vi "Send All HardWare Parameters Sending.vi"(0 "VISA resource name":refnum<visa-resource-name>="COM6", 5 "Corner Frecuency 1 [MHz]":u8=1 min=1 max=30 step=1, 7 "Corner Frecuency 2 [MHz]":u8=1 min=1 max=30 step=1, 9 "Gain VGA A (dB)":i8=-5 min=-5 max=45 step=1, 11 "Output Gain A":bool, 12 "Gain VGA B (dB)":i8=-5 min=-5 max=45 step=1, 13 "Output Gain B":bool) -> (10 "Coincidence Of Character":bool)   [LabVIEW 2011]
panel:
  in  "Numeric 3":fxp<+,12,12>
  out "String Sent DAC B":string
  out "Information Recieved DAC B":string
  out "Information Recieved DAC A":string
  out "String Sent DAC A":string
  in  "Numeric 2":fxp<+,12,12>
  out "Information Recieved PFVGA 2":string
  out "String Sent PFVGA 2":string
  out "Information Recieved PFVGA":string
  out "String Sent PFVGA":string
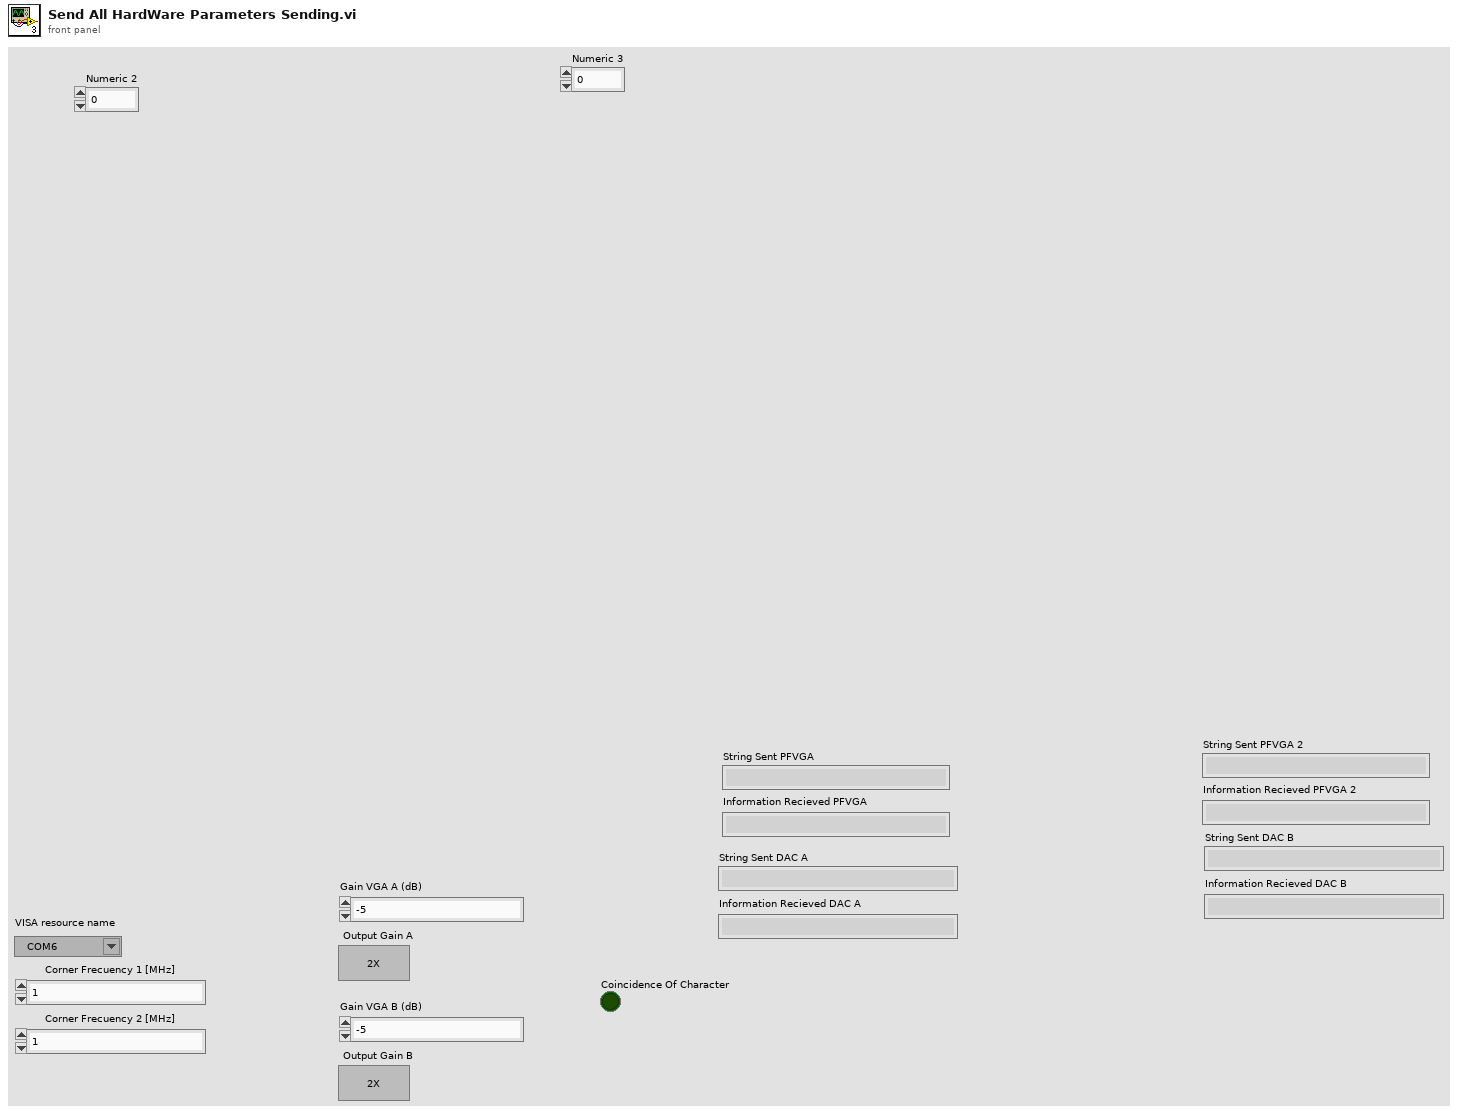
[diagram p1: front panel]
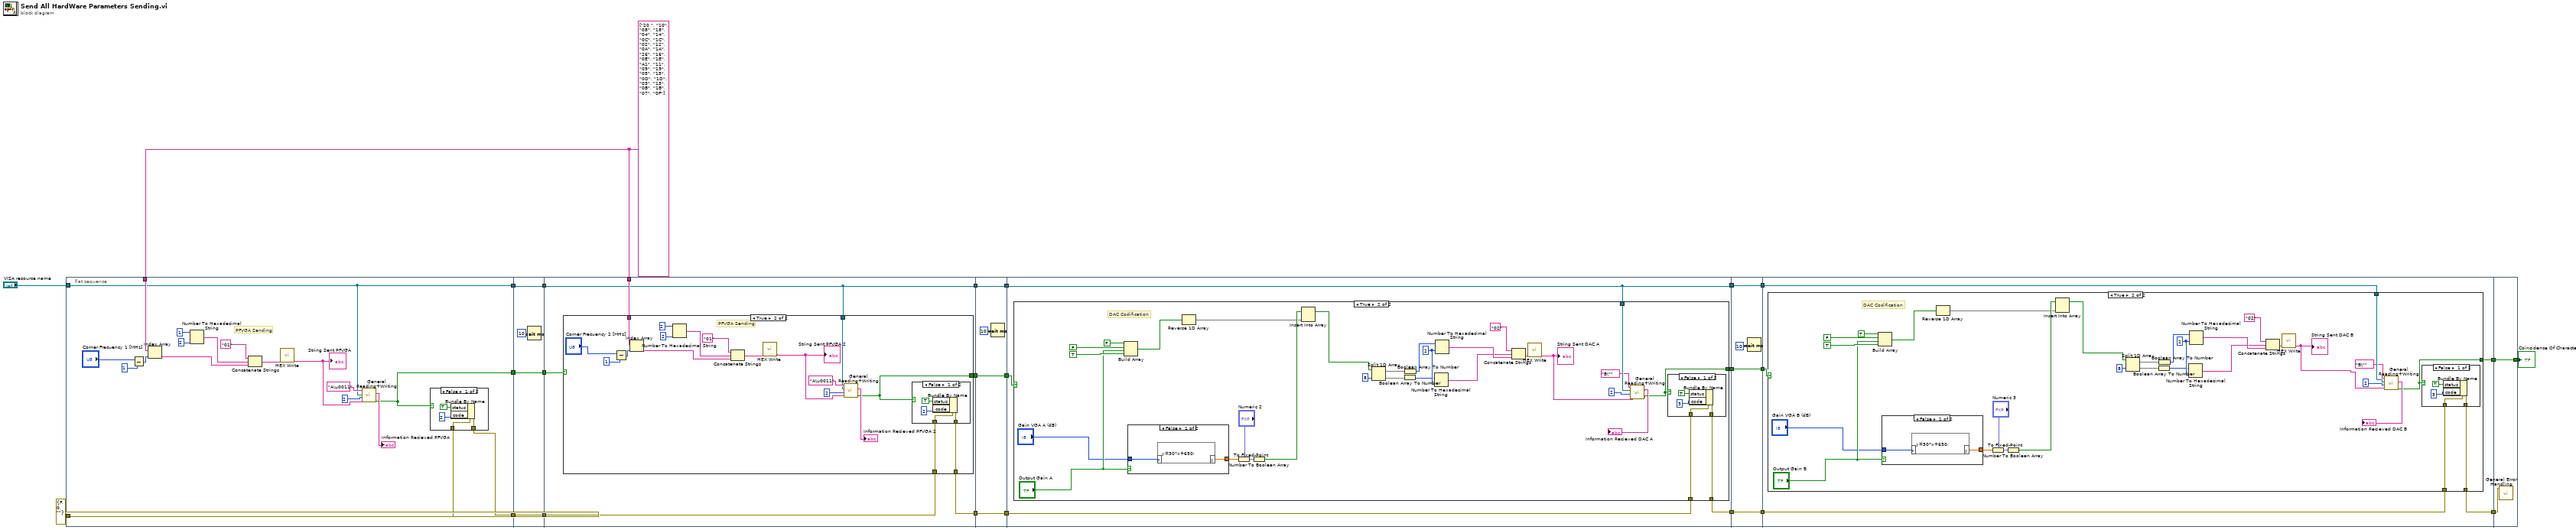
[diagram p0: block diagram]
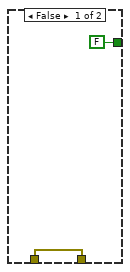
[diagram p3: hidden frame]
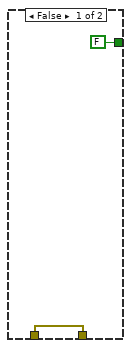
[diagram p5: hidden frame]
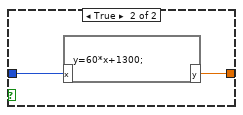
[diagram p7: hidden frame]
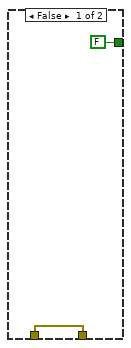
[diagram p8: hidden frame]
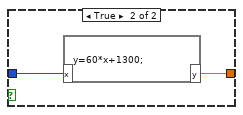
[diagram p10: hidden frame]
diagram:
  w23 = string[] ["20 ", "10", "08", "18", "04", "14", "0C", "1C", "02", "12", "0A", "1A", "26", "16", "0E", "1E", "A1", "11", "09", "19", "05", "15", "0D", "1D", "03", "13", "0B", "1B", "07", "0F"] ("Array")
  n1 = flat-sequence {
    tunnel: w23 -> [w33]
    tunnel: errorcluster {"status"=FALSE, "code"=0, "source"=""} ("error out") -> [w32]
    tunnel: [w31] -> w18
    tunnel: "VISA resource name" -> [w27]
    tunnel: [w25] -> w16
    tunnel: [w27] -> w14
    tunnel: w18 -> [w51]
    tunnel: [w51] -> w17
    tunnel: w16 -> [w50]
    tunnel: [w50] -> w15
    tunnel: w14 -> [w49]
    tunnel: [w49] -> w13
    tunnel: w17 -> [w56]
    tunnel: w23 -> [w57]
    tunnel: w15 -> [w54]
    tunnel: [w55] -> w12
    tunnel: w13 -> [w52]
    tunnel: [w53] -> w10
    tunnel: [w52] -> w8
    tunnel: w12 -> [w86]
    tunnel: [w86] -> w11
    tunnel: w10 -> [w85]
    tunnel: [w85] -> w9
    tunnel: w8 -> [w84]
    tunnel: [w84] -> w7
    tunnel: w11 -> [w90]
    tunnel: w9 -> [w91]
    tunnel: w7 -> [w88]
    tunnel: [w89] -> w6
    tunnel: [w88] -> w4
    tunnel: [w87] -> w2
    tunnel: w6 -> [w136]
    tunnel: [w136] -> w5
    tunnel: w4 -> [w135]
    tunnel: [w135] -> w3
    tunnel: w2 -> [w134]
    tunnel: [w134] -> w1
    tunnel: w5 -> [w141]
    tunnel: w3 -> [w139]
    tunnel: w1 -> [w138]
    tunnel: [w140] -> w20
    tunnel: [w137] -> w19
    tunnel: [w184] -> w21
    tunnel: w20 -> [w183]
    tunnel: w19 -> [w184]
    frame #0 {
      # "PFVGA Sending"
      n2 = Subtract(x="Corner Frecuency 1 [MHz]", y=u8 1) -> (x-y=w39:u8)
      n3 = Index Array(array=w33, index=w39) -> (element=w40:string)
      n4 = Number To Hexadecimal String(1:i16 2 ("width (-)"), 2:1 ("number")) -> (0:w34:string)
      n5 = Concatenate Strings("01" ("string"), w34, w40) -> (w37:string)
      n6 = call "HEX Write.vi"("String (Normal Display)"=w37) -> ("Result string (Hex Display)"=w29:string)  [unwired: 10 in]
      "String Sent PFVGA" <- w29
      n7 = call "General Reading+Writing.vi"("Write String"=w29, "Bytes to Read"=u32 2 ("Number bytes Read"), "VISA resource name"=w27, "String Seached"="A\u0011" ("search char")) -> ("Coincidence Of Character"=w25:bool, "read buffer"=→"Information Recieved PFVGA":string)  [unwired: 4 in, 2 out]
      n8 = case shown="False" w25 {
        tunnel: w32 -> [w44 w47]
        tunnel: [w43 w47] -> w31
        frame False {
          n9 = Bundle By Name(cluster=w44, "status"=TRUE, "code"=2) -> (w43:errorcluster)
        }
        frame True {
        }
      }
    }
    frame #1 {
      n10 = Wait (ms)(milliseconds to wait=u32 10) -> ()  [unwired: 1 out]
    }
    frame #2 {
      n11 = case shown="True" w54 {
        tunnel: w57 -> [_ w68]
        tunnel: w56 -> [w59 w67]
        tunnel: [w59 w66] -> w55
        tunnel: [FALSE ("Coincidence Of Character") w60] -> w53
        tunnel: w52 -> [_ w63]
        frame False {
        }
        frame True {
          # "PFVGA Sending"
          n12 = Subtract(x="Corner Frecuency 2 [MHz]", y=u8 1) -> (x-y=w72:u8)
          n13 = Index Array(array=w68, index=w72) -> (element=w71:string)
          n14 = Number To Hexadecimal String(1:i16 2 ("width (-)"), 2:2 ("number")) -> (0:w77:string)
          n15 = Concatenate Strings("01" ("string"), w77, w71) -> (w74:string)
          n16 = call "HEX Write.vi"("String (Normal Display)"=w74) -> ("Result string (Hex Display)"=w65:string)  [unwired: 10 in]
          "String Sent PFVGA 2" <- w65
          n17 = call "General Reading+Writing.vi"("Write String"=w65, "Bytes to Read"=u32 2 ("Number bytes Read"), "VISA resource name"=w63, "String Seached"="A\u0011" ("search char")) -> ("Coincidence Of Character"=w60:bool, "read buffer"=→"Information Recieved PFVGA 2":string)  [unwired: 4 in, 2 out]
          n18 = case shown="False" w60 {
            tunnel: w67 -> [w79 w82]
            tunnel: [w78 w82] -> w66
            frame False {
              n19 = Bundle By Name(cluster=w79, "status"=TRUE, "code"=2) -> (w78:errorcluster)
            }
            frame True {
            }
          }
        }
      }
    }
    frame #3 {
      n20 = Wait (ms)(milliseconds to wait=u32 10) -> ()  [unwired: 1 out]
    }
    frame #4 {
      n21 = case shown="True" w91 {
        tunnel: w90 -> [w93 w101]
        tunnel: w88 -> [_ w99]
        tunnel: [w93 w100] -> w89
        tunnel: [FALSE ("Coincidence Of Character") w94] -> w87
        frame False {
        }
        frame True {
          w123 = i16 2 ("width (-)")
          # "DAC Codification"
          n22 = Build Array(FALSE ("element"), FALSE ("A/B"), "Output Gain A", TRUE ("element")) -> (w111:bool[])
          n23 = case shown="False" "Output Gain A" {
            tunnel: "Gain VGA A (dB)" -> [w130 w132]
            tunnel: [w129 w131] -> w112
            frame False {
              n24 = formula code="y=30*x+650;"("x"=w130) -> ("y"=w129:dbl)
            }
            frame True {
              n25 = formula code="y=60*x+1300;"("x"=w132) -> ("y"=w131:dbl)
            }
          }
          n26 = Reverse 1D Array(array=w111) -> (reversed array=w109:bool[])
          n27 = To Fixed-Point(fixed-point type="Numeric 2", number=w112) -> (fixed-point=w115:fxp<+,12,12>)
          n28 = Number To Boolean Array(number=w115) -> (Boolean array=w110:bool[])
          n29 = Insert Into Array(array=w110, new element=w109) -> (w119:bool[])  [unwired: 1 in]
          n30 = Split 1D Array(array=w119, index=8) -> (first subarray=w117:bool[], second subarray=w118:bool[])
          n31 = Boolean Array To Number(Boolean array=w118) -> (number=w121:u32)
          n32 = Boolean Array To Number(Boolean array=w117) -> (number=w122:u32)
          n33 = Number To Hexadecimal String(1:w123, 2:w121) -> (0:w107:string)
          n34 = Number To Hexadecimal String(1:w123, 2:w122) -> (0:w108:string)
          n35 = Concatenate Strings("02" ("string"), w107, w108) -> (w106:string)
          n36 = call "HEX Write.vi"("String (Normal Display)"=w106) -> ("Result string (Hex Display)"=w96:string)  [unwired: 10 in]
          "String Sent DAC A" <- w96
          n37 = call "General Reading+Writing.vi"("Write String"=w96, "Bytes to Read"=u32 2 ("Number bytes Read"), "VISA resource name"=w99, "String Seached"="B\"" ("search char")) -> ("Coincidence Of Character"=w94:bool, "read buffer"=→"Information Recieved DAC A":string)  [unwired: 4 in, 2 out]
          n38 = case shown="False" w94 {
            tunnel: w101 -> [w125 w128]
            tunnel: [w124 w128] -> w100
            frame False {
              n39 = Bundle By Name(cluster=w125, "status"=TRUE, "code"=3) -> (w124:errorcluster)
            }
            frame True {
            }
          }
        }
      }
    }
    frame #5 {
      n40 = Wait (ms)(milliseconds to wait=u32 10) -> ()  [unwired: 1 out]
    }
    frame #6 {
      n41 = case shown="True" w138 {
        tunnel: w141 -> [w143 w151]
        tunnel: w139 -> [_ w145]
        tunnel: [w143 w150] -> w140
        tunnel: [FALSE ("Coincidence Of Character") w148] -> w137
        frame False {
        }
        frame True {
          w173 = i16 2 ("width (-)")
          # "DAC Codification"
          n42 = Build Array(TRUE ("element"), FALSE ("A/B"), "Output Gain B", TRUE ("element")) -> (w161:bool[])
          n43 = case shown="False" "Output Gain B" {
            tunnel: "Gain VGA B (dB)" -> [w180 w182]
            tunnel: [w179 w181] -> w162
            frame False {
              n44 = formula code="y=30*x+650;"("x"=w180) -> ("y"=w179:dbl)
            }
            frame True {
              n45 = formula code="y=60*x+1300;"("x"=w182) -> ("y"=w181:dbl)
            }
          }
          n46 = Reverse 1D Array(array=w161) -> (reversed array=w159:bool[])
          n47 = To Fixed-Point(fixed-point type="Numeric 3", number=w162) -> (fixed-point=w165:fxp<+,12,12>)
          n48 = Number To Boolean Array(number=w165) -> (Boolean array=w160:bool[])
          n49 = Insert Into Array(array=w160, new element=w159) -> (w169:bool[])  [unwired: 1 in]
          n50 = Split 1D Array(array=w169, index=8) -> (first subarray=w167:bool[], second subarray=w168:bool[])
          n51 = Boolean Array To Number(Boolean array=w168) -> (number=w171:u32)
          n52 = Boolean Array To Number(Boolean array=w167) -> (number=w172:u32)
          n53 = Number To Hexadecimal String(1:w173, 2:w171) -> (0:w157:string)
          n54 = Number To Hexadecimal String(1:w173, 2:w172) -> (0:w158:string)
          n55 = Concatenate Strings("02" ("string"), w157, w158) -> (w156:string)
          n56 = call "HEX Write.vi"("String (Normal Display)"=w156) -> ("Result string (Hex Display)"=w147:string)  [unwired: 10 in]
          "String Sent DAC B" <- w147
          n57 = call "General Reading+Writing.vi"("Write String"=w147, "Bytes to Read"=u32 2 ("Number bytes Read"), "VISA resource name"=w145, "String Seached"="B\"" ("search char")) -> ("Coincidence Of Character"=w148:bool, "read buffer"=→"Information Recieved DAC B":string)  [unwired: 4 in, 2 out]
          n58 = case shown="False" w148 {
            tunnel: w151 -> [w175 w178]
            tunnel: [w174 w178] -> w150
            frame False {
              n59 = Bundle By Name(cluster=w175, "status"=TRUE, "code"=3) -> (w174:errorcluster)
            }
            frame True {
            }
          }
        }
      }
    }
    frame #7 {
      n60 = call "General Error Handling.vi"("error IO"=w183) -> ()  [unwired: 11 in]
    }
  }
  "Coincidence Of Character" <- w21
